vi "Discover NFA Model.vi"(10 "Model In":string) -> (2 "selection":bool)   [LabVIEW 2018]
panel:
  out "size(s)":i32
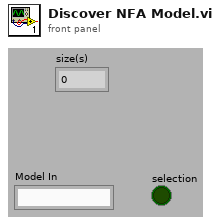
[diagram p1: front panel]
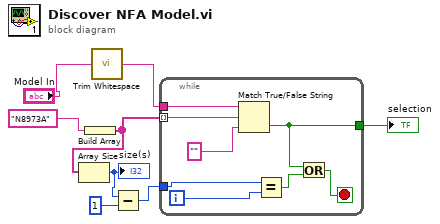
[diagram p0: block diagram]
diagram:
  n1 = Build Array("N8973A" ("true string")) -> (w6:string[])
  n2 = Array Size(array=w6) -> (size(s)=w5:i32)
  "size(s)" <- w5
  n3 = call <vilib>:"Trim Whitespace.vi"("string"="Model In") -> ("trimmed string"=w1:string)  [unwired: 1 in]
  n4 = Subtract(x=w5, y=1) -> (x-y=w3:i32)
  n5 = while {
    tunnel: w6 -> [w15] mode=indexing
    tunnel: w1 -> [w14]
    tunnel: [w13] -> w7
    tunnel: w3 -> [w9]
    i -> [w10]
    stop <- w12 stop-if-true
    n6 = Match True/False String(2:"" ("false string"), 3:w15, 4:w14) -> (0:w13:bool)  [unwired: 1 out]
    n7 = Equal?(x=w9, y=w10) -> (x = y?=w11:bool)
    n8 = Or(x=w13, y=w11) -> (x .or. y?=w12:bool)
  }
  "selection" <- w7
